vi "Action Save Curve to Flash.vi"(0 "VISA resource name":refnum<visa-resource-name>, 7 "Save Curve to Flash (T: Save)":bool=TRUE, 11 "error in (no error)":errorcluster) -> (4 "VISA resource name out":refnum<visa-resource-name>, 15 "error out":errorcluster)   [LabVIEW 2019, in "Lake Shore Cryotronics 340.lvlib"]
doc: "This vi updates the Curve Flash with the current user curves. May take several seconds; use the Status Busy.vi to determine when complete."
uses:
  Lake Shore Cryotronics 340.lvlib
panel:
  # "Save Curve\nDon't Save Curve"
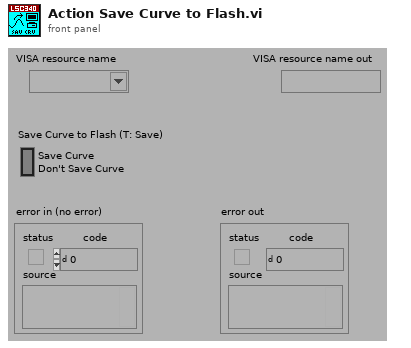
[diagram p1: front panel]
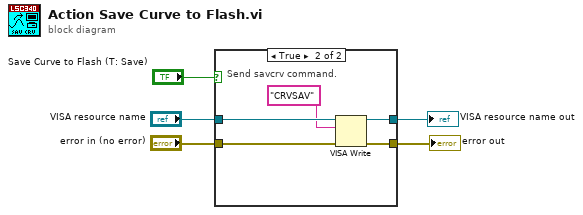
[diagram p0: block diagram]
diagram:
  n1 = case shown="True" "Save Curve to Flash (T: Save)" {
    tunnel: "error in (no error)" -> [w6 w9]
    tunnel: "VISA resource name" -> [w7 w12]
    tunnel: [w7 w11] -> w1
    tunnel: [w6 w10] -> w2
    frame False {
      # "Do not save curve."
    }
    frame True {
      # "Send savcrv command."
      n2 = VISA Write(VISA resource name=w12, write buffer="CRVSAV", error in (no error)=w9) -> (VISA resource name out=w11:refnum<visa-resource-name>, error out=w10:errorcluster)  [unwired: 1 out]
    }
  }
  "error out" <- w2
  "VISA resource name out" <- w1
